vi "LWXPS_GetAccParams.vi"(0 "XPS Reference IN":refnum<k24>, 5 "LabVIEW error IN":errorcluster) -> (12 "XPS Reference OUT":refnum<k24>, 13 "LabVIEW error OUT":errorcluster, 14 "Returned error code":i32, 15 "X Acceleration time in ms":i32, 16 "X Smooth factor in ms":i32, 17 "Y Acceleration time in ms":i32, 18 "Y Smooth factor in ms":i32, 19 "XPS Error String":string)   [LabVIEW 2014]
uses:
  D:/XPSQ8_LabView_Library/Development/Source/Dll/Newport.XPS.CommandInterface.dll
  Dll/Newport.XPS.CommandInterface.dll
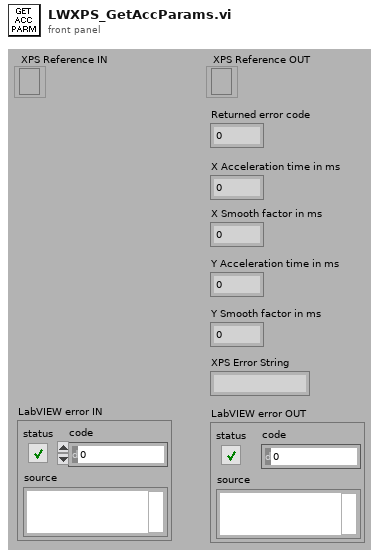
[diagram p1: front panel]
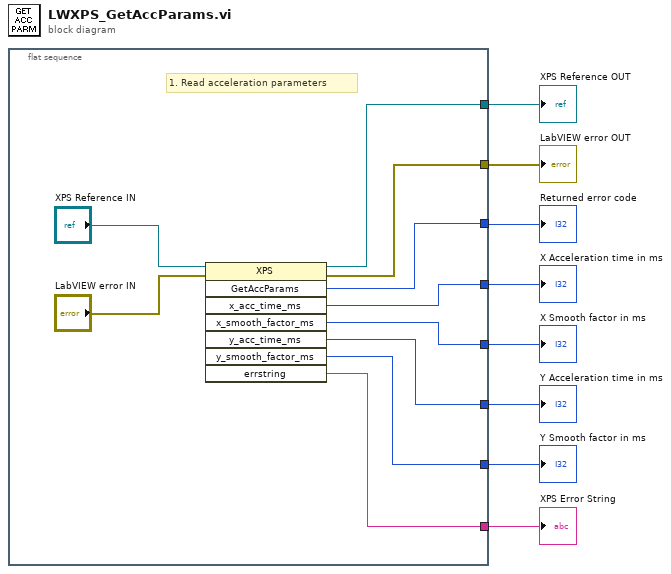
[diagram p0: block diagram]
diagram:
  n1 = flat-sequence {
    tunnel: [w17] -> w5
    tunnel: [w16] -> w8
    tunnel: [w15] -> w7
    tunnel: [w14] -> w6
    tunnel: [w12] -> w4
    tunnel: [w11] -> w3
    tunnel: [w10] -> w1
    tunnel: [w9] -> w2
    frame #0 {
      # "1. Read acceleration parameters"
      n2 = invoke class="XPS" method="GetAccParams"(reference="XPS Reference IN", error in="LabVIEW error IN") -> (reference out=w16:refnum<k24>, error out=w15:errorcluster, "GetAccParams"=w14:i32, "x_acc_time_ms"=w17:i32, "x_smooth_factor_ms"=w12:i32, "y_acc_time_ms"=w11:i32, "y_smooth_factor_ms"=w10:i32, "errstring"=w9:string)  [unwired: 6 in]
    }
  }
  "XPS Error String" <- w2
  "XPS Reference OUT" <- w8
  "LabVIEW error OUT" <- w7
  "Returned error code" <- w6
  "X Acceleration time in ms" <- w5
  "X Smooth factor in ms" <- w4
  "Y Acceleration time in ms" <- w3
  "Y Smooth factor in ms" <- w1
